vi "Read Ready_.vi"(8 "error in (no error)":errorcluster, 11 "Sequence State Msg in":refnum<class "Sequence State Msg.lvclass">) -> (0 "error out":errorcluster, 2 "Ready?":bool, 3 "Sequence State Msg out":refnum<class "Sequence State Msg.lvclass">)   [LabVIEW 2014, in "HIJ Vision Camera App.lvlib" / "Sequence State Msg.lvclass"]
uses:
  Sequence State Msg.lvclass
  Sequence State Msg.lvclass/Sequence State Msg.ctl
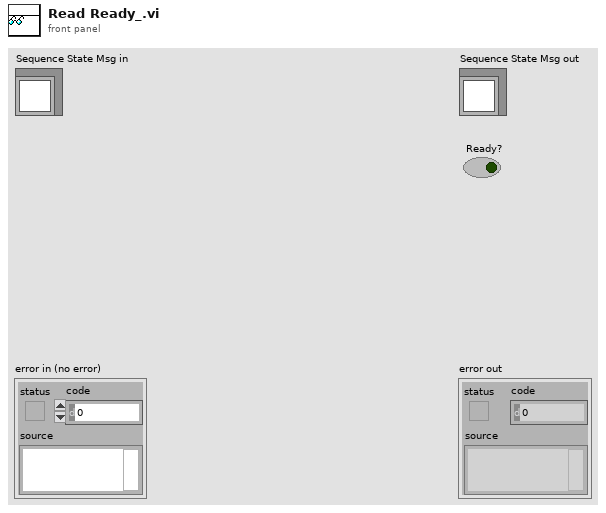
[diagram p1: front panel]
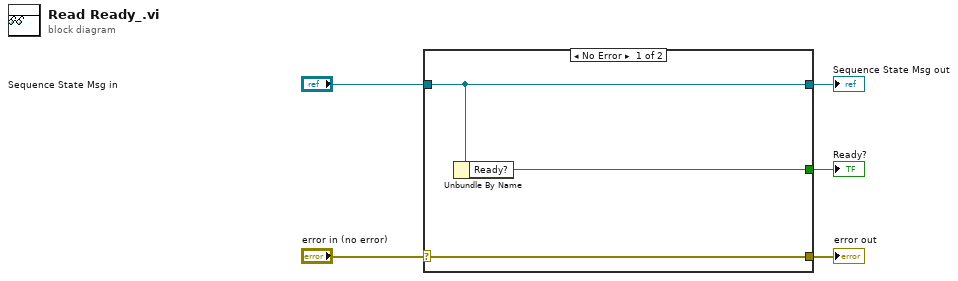
[diagram p0: block diagram]
diagram:
  n1 = case shown="No Error" "error in (no error)" {
    selector: "error in (no error)" -> [w8 w9]
    tunnel: [w8 w9] -> w4
    tunnel: [w7 w10] -> w2
    tunnel: "Sequence State Msg in" -> [w7 w10]
    tunnel: [w6 _] -> w1
    frame No Error {
      n2 = Unbundle By Name(w7) -> ("Ready?"=w6:bool)
    }
    frame Error {
    }
  }
  "error out" <- w4
  "Sequence State Msg out" <- w2
  "Ready?" <- w1
